vi "Test_API_LogItemDataSource_EventSourceMatch.vi"(8 "error in (no error)":errorcluster, 11 "TestCase in":refnum<class "TestLocalLogInstance.lvclass">) -> (0 "error out":errorcluster, 3 "TestCase out":refnum<class "TestLocalLogInstance.lvclass">)   [LabVIEW 2017, in "TestLocalLogInstance.lvclass"]
uses:
  TestLocalLogInstance.lvclass
  Source/Composed Log/Types/Log Level.ctl
  Source/Composed Log/LoggerReference/LoggerReference.lvclass/LoggerReference.ctl
  Source/LVQueue Sink/LVQueue Sink.lvclass/LVQueue Sink.ctl
  93e12b67-f617-4ac9-a0f1-5371faa10247.vi
  Source/Composed Log/LoggerReference/Return Aggregate Queues.vi
  Source/Composed Log/LoggerReference/Add Aggregate Log.vi
  93e12b67-f617-4ac9-a0f1-5371faa10247.vi/2c634974-dd49-458f-9370-0b106b71e0c8.vi
  Source/Composed Log/LoggerReference/Log.vi
  Source/Composed Log/LoggerReference/Send Add Sink.vi
  Source/Composed Log/LoggerReference/Remove Stale Logs.vi
  Source/LVQueue Sink/LVQueue Sink.lvclass
  C:/CS/Internal/LabVIEW/Logger/Source/Composed Log/Log Sink/Log Sink.lvclass
  Source/Composed Log/Application Logger/Launch Worker Loop.vi
  Source/Composed Log/LoggerReference/Initialize Logger Instance.vi
  Source/Composed Log/LoggerReference/LoggerReference.lvclass
  Source/Composed Log/IErrorFormat/IErrorFormat.lvclass
  Source/Composed Log/Log Sink/Log Sink.lvclass
  <vilib>/addons/_JKI Toolkits/VI Tester/TestCase.llb/TestCase.lvclass
  Source/Composed Log/Composed Log.lvlib
  C:/Program Files (x86)/National Instruments/LabVIEW 2017/vi.lib/addons/_JKI Toolkits/VI Tester/TestCase.llb/TestCase.lvclass
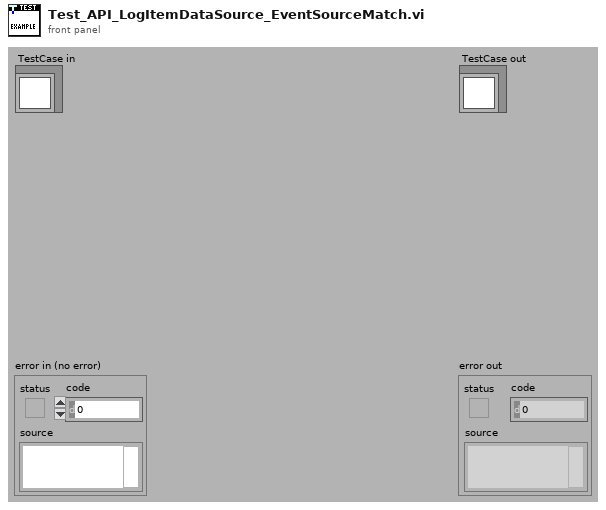
[diagram p1: front panel]
types:
  T1 = typedef "Composed Log.lvlib/Log Level.ctl" = enum16{"Debug", "Info", "Warning", "Error", "Critical"}
  T2 = typedef "Composed Log.lvlib/Log Packet.ctl" = cluster{"Data To Log":string, "Source":string, "Event Level":T1, "Event Time":timestamp}
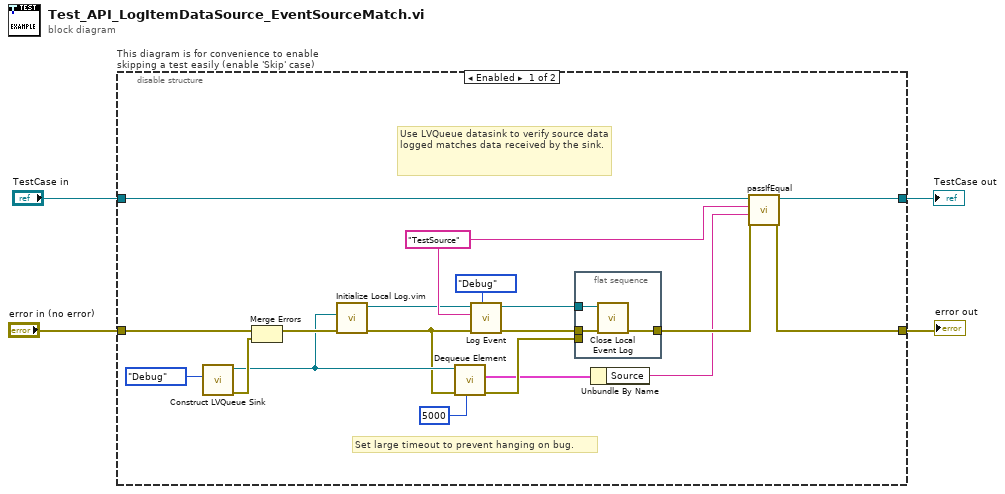
[diagram p0: block diagram]
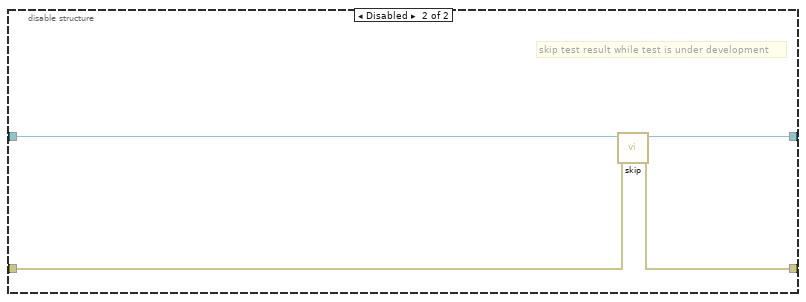
[diagram p2: hidden frame]
diagram:
  n1 = disable-structure "This diagram is for convenience to enable skipping a test easily (enable 'Skip' case)" shown="Enabled" {
    disable-tunnel: "TestCase in" -> [w21 w30]
    disable-tunnel: [w22 w28] -> w1
    disable-tunnel: [w20 w29] -> w3
    disable-tunnel: "error in (no error)" -> [w23 w27]
    frame Enabled {
      w10 = "TestSource" ("Data To Log")
      # "Set large timeout to prevent hanging on bug."
      # "Use LVQueue datasink to verify source data logged matches data received by the sink."
      n2 = call "Construct LVQueue Sink.vi"("LogLevel"=Log_Level."Debug") -> ("error out"=w11:errorcluster, "LVQueue Sink out"=w8:refnum<class "LVQueue Sink.lvclass">)  [unwired: 9 in]
      n3 = Merge Errors(w23, w11) -> (w9:errorcluster)
      n4 = call "Initialize Local Log.vim"("error in (no error)"=w9, "Startup Sink(s)"=w8) -> ("error out"=w7:errorcluster, "Log Instance Reference"=w6:refnum<class "LoggerReference.lvclass">)  [unwired: 7 in, 1 out]
      n5 = call "Dequeue Element.vi"("timeout in ms (-1)"=5000, "error in (no error)"=w7, "LVQueue Sink in"=w8) -> ("error out"=w16:errorcluster, "Log Packet"=w13:T2)  [unwired: 5 in, 2 out]
      n6 = call "Log Event.vi"("Event Level"=Log_Level."Debug", "error in (no error)"=w7, "SourceID"=w10, "Log Instance"=w6) -> ("error out"=w17:errorcluster, "Log Instance Out"=w5:refnum<class "LoggerReference.lvclass">)  [unwired: 6 in]
      n7 = flat-sequence {
        tunnel: [w25] -> w14
        tunnel: w17 -> [w26]
        tunnel: w16 -> [_]
        tunnel: w5 -> [w24]
        frame #0 {
          n8 = call "Close Local Event Log.vi"("error in (no error)"=w26, "Log Instance"=w24) -> ("error out"=w25:errorcluster)  [unwired: 9 in]
        }
      }
      n9 = Unbundle By Name(w13) -> ("Source"=w12:string)
      n10 = call-dynamic "passIfEqual.vi"("error in (no error)"=w14, "y"=w12, "x"=w10, "TestCase in"=w21) -> ("error out"=w20:errorcluster, "TestCase out"=w22:refnum<class "TestLocalLogInstance.lvclass">)  [unwired: 6 in]
    }
    frame Disabled {
      # "skip test result while test is under development"
      n11 = call <vilib>:"skip.vi"("error in (no error)"=w27, "TestCase in"=w30) -> ("error out"=w29:errorcluster, "TestCase out"=w28:refnum<class "TestLocalLogInstance.lvclass">)  [unwired: 8 in]
    }
  }
  "error out" <- w3
  "TestCase out" <- w1
